vi "MotionProfileGeneratorPosition.vi"(1 "Trajectory Point Interval (ms)":i32, 2 "Velocity":dbl, 3 "Previous Position":dbl, 4 "Previous Velocity":dbl) -> (0 "Position":dbl)   [LabVIEW 2017]
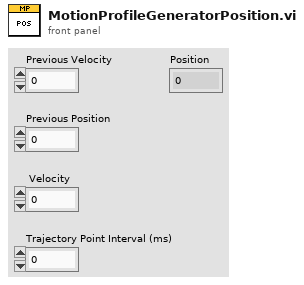
[diagram p1: front panel]
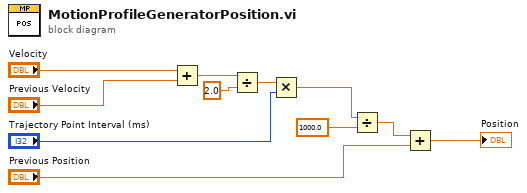
[diagram p0: block diagram]
diagram:
  n1 = Add(x="Velocity", y="Previous Velocity") -> (x+y=w10:dbl)
  n2 = Divide(x=w10, y=2.0) -> (x/y=w7:dbl)
  n3 = Multiply(x=w7, y="Trajectory Point Interval (ms)") -> (x*y=w6:dbl)
  n4 = Divide(x=w6, y=1000.0) -> (x/y=w8:dbl)
  n5 = Add(x=w8, y="Previous Position") -> (x+y=→"Position":dbl)
